vi "Read.vi"   [LabVIEW 2015, in "Agilent 3446X Series1.lvlib"]
doc: "Allows users to read one or more measurements from the DMM."
uses:
  Agilent 3446X Series1.lvlib
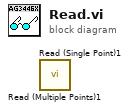
[diagram p0: block diagram]
diagram:
  n1 = call "Read (Multiple Points)1.vi"() -> ()  [unwired: 9 in, 3 out]
  n2 = call "Read (Single Point)1.vi"() -> ()  [unwired: 9 in, 3 out]
